vi "CmdExe.Get Processes with Kill Option.vi"(6 "Kill Only 1 Instance":bool=TRUE, 7 "Name Contains":bool, 8 "Error In":errorcluster, 9 "Kill Task":bool, 10 "Process Name":string) -> (0 "Error Out":errorcluster, 1 "Task Killed":bool, 2 "Tasks":string[][](table), 3 "Is Running":bool)   [LabVIEW 2024]
uses:
  <vilib>/Utility/error.llb/Trim Whitespace One-Sided.vi
  <vilib>/KATE/Strings/String Utils.lvlib
panel:
  in  "Tab Control":enum32{"Table", "STDIO"}(tab)
  out "standard output":string
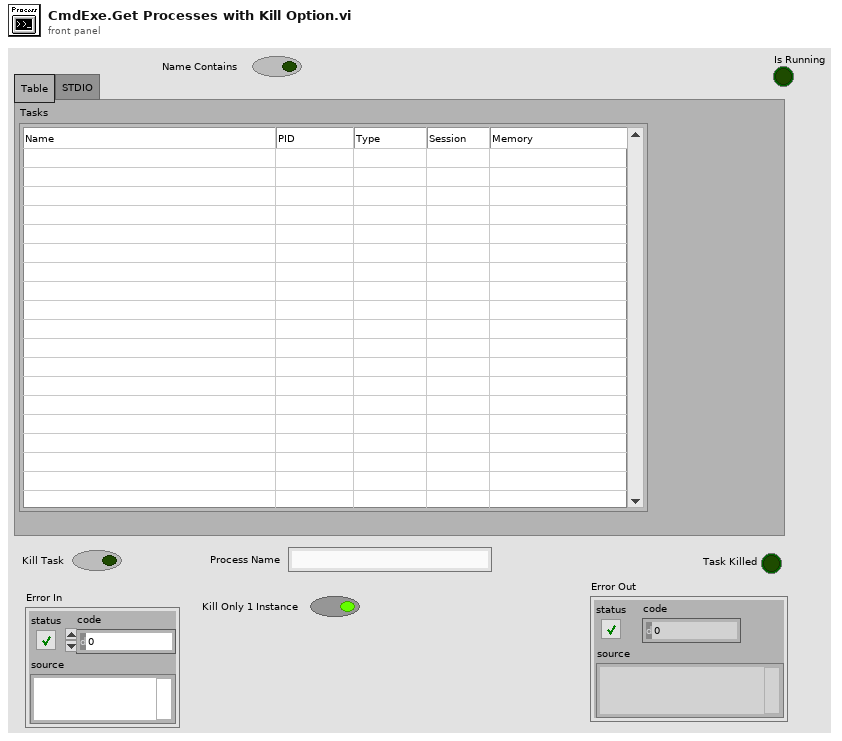
[diagram p1: front panel]
types:
  T1 = cluster{"Stdout":string, "Tasks":string[][], "Index":i32, "PIDs":string[]}
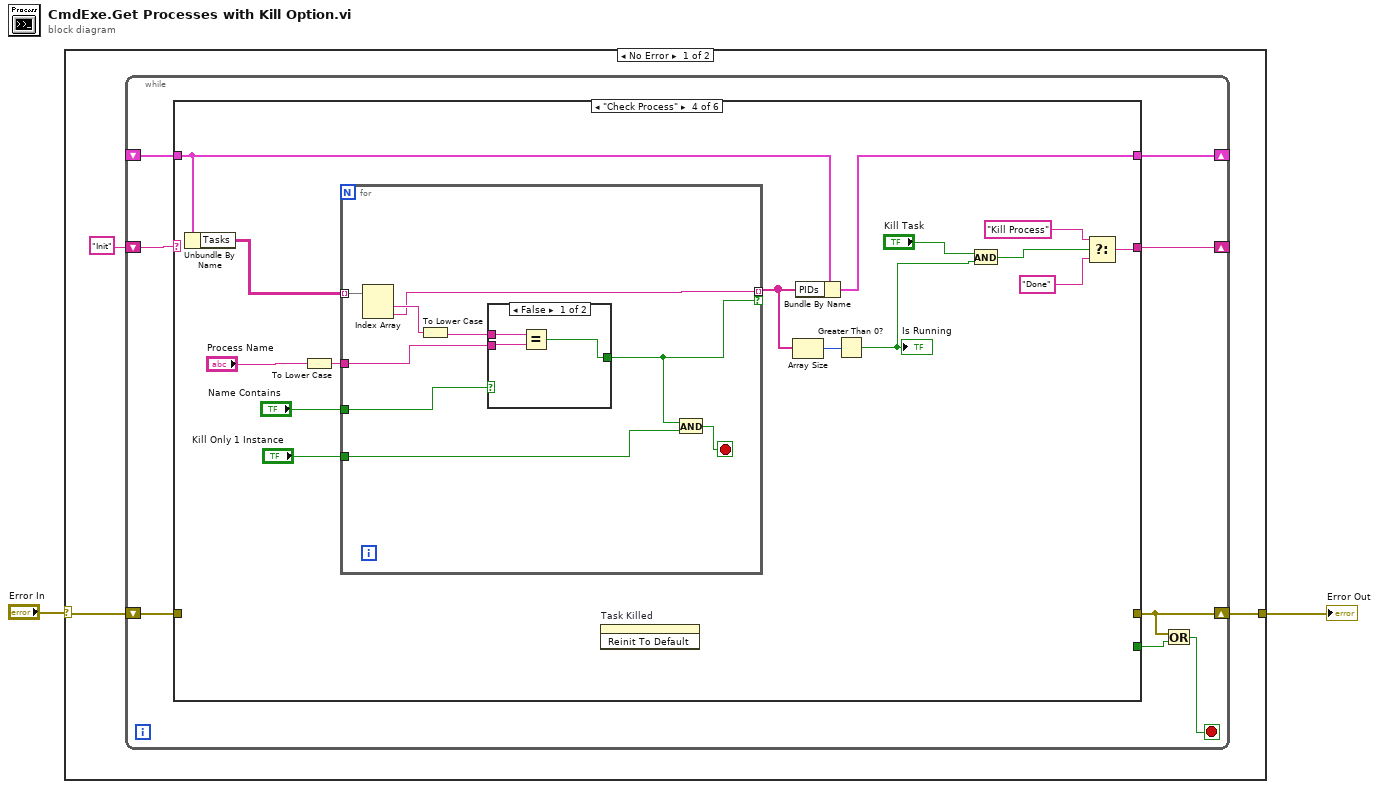
[diagram p0: block diagram]
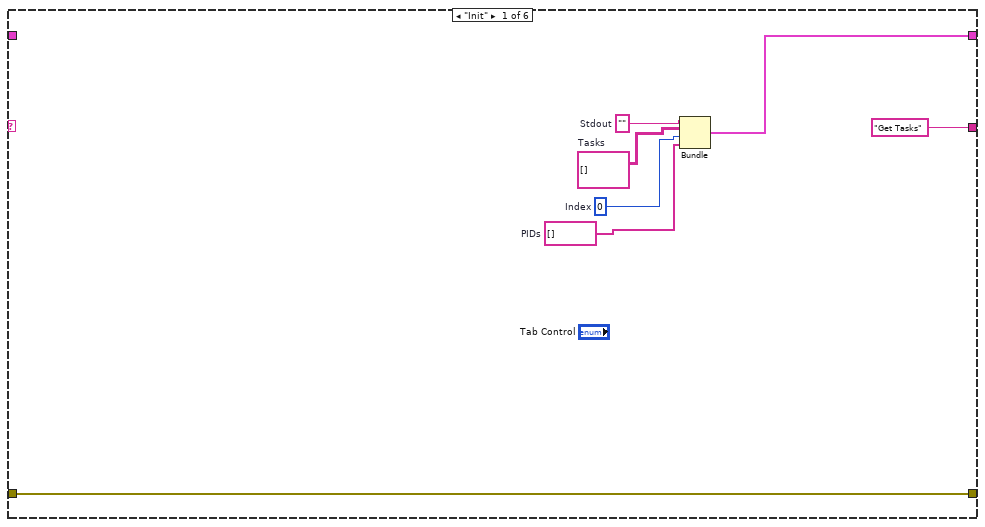
[diagram p2: hidden frame]
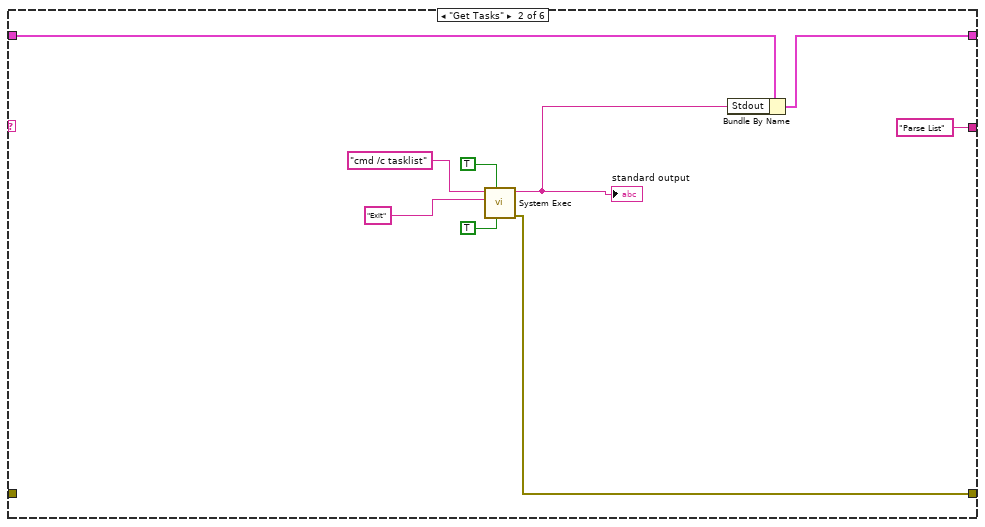
[diagram p3: hidden frame]
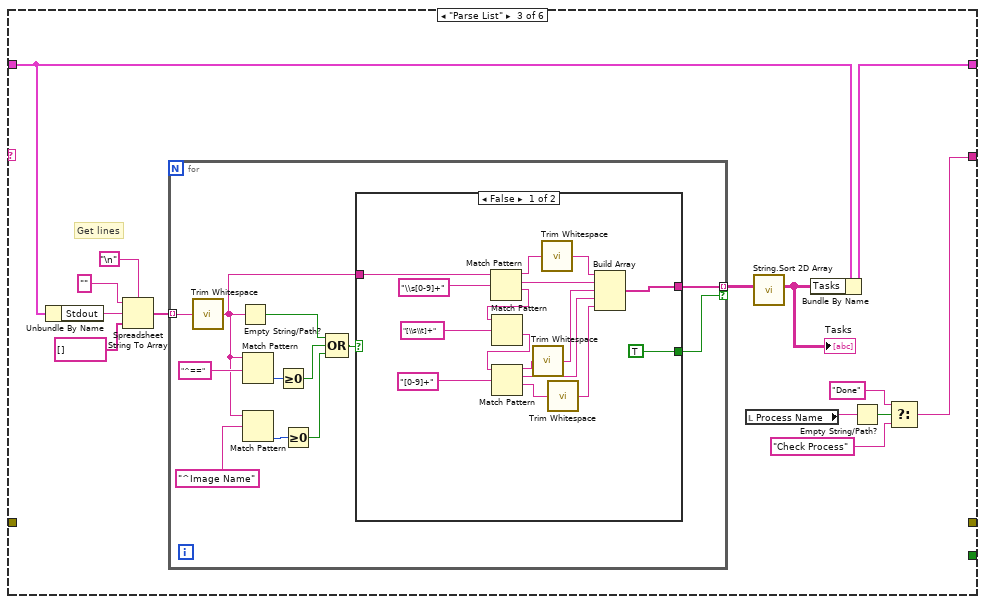
[diagram p4: hidden frame]
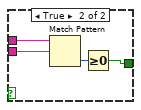
[diagram p6: hidden frame]
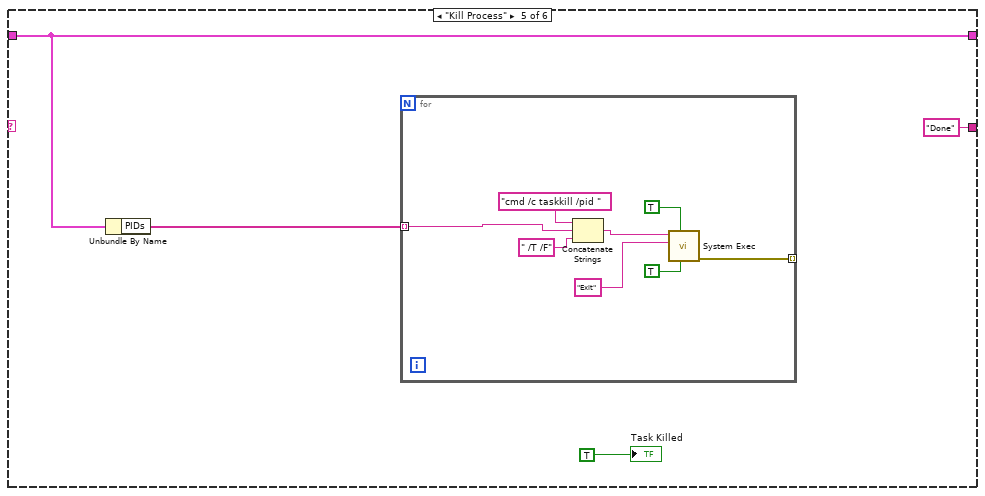
[diagram p7: hidden frame]
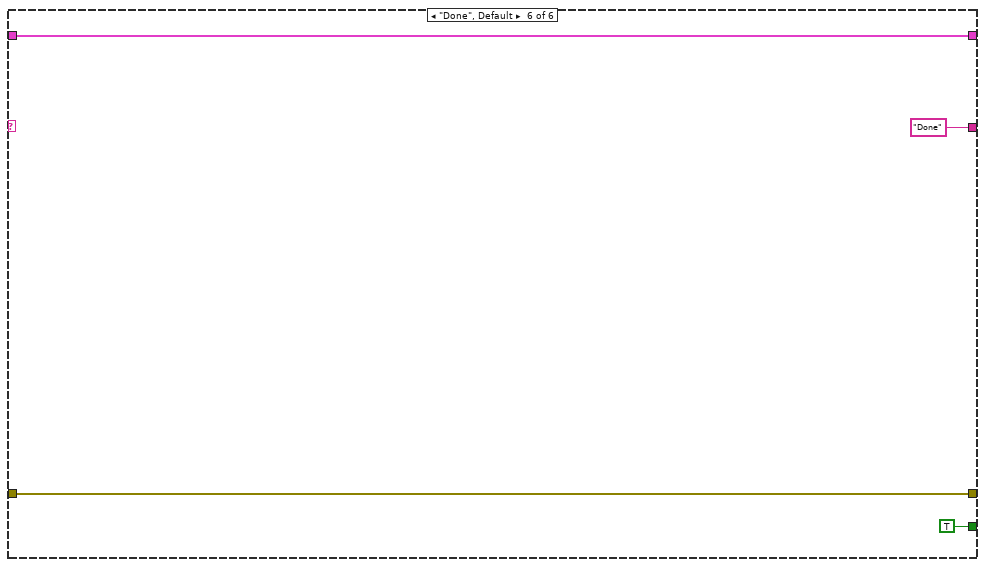
[diagram p8: hidden frame]
diagram:
  n1 = case shown="No Error" "Error In" {
    selector: "Error In" -> [w3 w119]
    tunnel: [w4 w119] -> w2
    frame No Error {
      n2 = while {
        shift-right: [w8] -> _
        shift-left: _ -> [w13]
        shift-right: [w7] -> _
        shift-left: "Init" -> [w9]
        shift-right: [w11] -> w4
        shift-left: w3 -> [w12]
        stop <- w10 stop-if-true
        n3 = case shown="\"Check Process\"" w9 {
          tunnel: w13 -> [_ w28 w41 w85 w105 w118]
          tunnel: w12 -> [w20 _ _ _ _ w116]
          tunnel: [w20 w23 _ _ _ w116] -> w11
          tunnel: [w18 w27 w43 w84 w105 w118] -> w8
          tunnel: ["Get Tasks" "Parse List" w30 w81 "Done" "Done"] -> w7
          tunnel: [_ _ _ _ _ TRUE] -> w6
          frame "Init" {
            w14 = string[] []  # PIDs
            w15 = 0  # Index
            w16 = string[][] []  # Tasks
            w19 = ""  # Stdout
            n4 = Bundle("Stdout"=w19, "Tasks"=w16, "Index"=w15, "PIDs"=w14) -> (w18:T1)  [unwired: 1 in]
          }
          frame "Get Tasks" {
            n5 = call <vilib>:"System Exec.vi"("run minimized? (F)"=TRUE, "wait until completion? (T)"=TRUE, "standard input"="Exit", "command line"="cmd /c tasklist" ("name or relative path")) -> ("error out"=w23:errorcluster, "standard output"=w24:string)  [unwired: 4 in, 2 out]
            "standard output" <- w24
            n6 = Bundle By Name(cluster=w28, "Stdout"=w24) -> (w27:T1)
          }
          frame "Parse List" {
            # "Get lines"
            n7 = Unbundle By Name(w41) -> ("Stdout"=w40:string)
            n8 = Spreadsheet String To Array(delimiter (Tab)="\n", format string="", spreadsheet string=w40, array type (2D Dbl)=string[] [] ("Tasks")) -> (array=w38:string[])
            n9 = for {
              tunnel: w38 -> [w55] mode=indexing
              tunnel: [w49] -> w36 mode=indexing if=w48
              n10 = call <vilib>:"Trim Whitespace.vi"("string"=w55) -> ("trimmed string"=w44:string)  [unwired: 1 in]
              n11 = Empty String/Path?(string/path=w44) -> (empty?=w51:bool)
              n12 = Match Pattern(string=w44, regular expression="^==" ("delimiter (Tab)")) -> (offset past match=w53:i32)  [unwired: 1 in, 3 out]
              n13 = Match Pattern(string=w44, regular expression="^Image Name" ("delimiter (Tab)")) -> (offset past match=w46:i32)  [unwired: 1 in, 3 out]
              n14 = Greater Or Equal To 0?(x=w53) -> (x >= 0?=w52:bool)
              n15 = Greater Or Equal To 0?(x=w46) -> (x >= 0?=w45:bool)
              n16 = Compound Arithmetic op=OR(w51, w52, w45) -> (w50:bool)
              n17 = case shown="False" w50 {
                tunnel: w44 -> [w71 _]
                tunnel: [w68 _] -> w49
                tunnel: [TRUE _] -> w48
                frame False {
                  n18 = Match Pattern(string=w71, regular expression="\\s[0-9]+" ("delimiter (Tab)")) -> (before substring=w58:string, match substring=w62:string, after substring=w70:string)  [unwired: 1 in, 1 out]
                  n19 = Match Pattern(string=w70, regular expression="[\\s\\t]+" ("delimiter (Tab)")) -> (after substring=w69:string)  [unwired: 1 in, 3 out]
                  n20 = Match Pattern(string=w69, regular expression="[0-9]+" ("delimiter (Tab)")) -> (before substring=w57:string, match substring=w61:string, after substring=w63:string)  [unwired: 1 in, 1 out]
                  n21 = call <vilib>:"Trim Whitespace.vi"("string"=w57) -> ("trimmed string"=w56:string)  [unwired: 1 in]
                  n22 = call <vilib>:"Trim Whitespace.vi"("string"=w58) -> ("trimmed string"=w59:string)  [unwired: 1 in]
                  n23 = call <vilib>:"Trim Whitespace.vi"("string"=w63) -> ("trimmed string"=w60:string)  [unwired: 1 in]
                  n24 = Build Array(w59, w62, w56, w61, w60) -> (w68:string[])
                }
                frame True {
                }
              }
            }
            n25 = local read "Process Name"() -> (w33:string)
            n26 = call <vilib>:"String.Sort 2D Array.vi"("Array In"=w36) -> ("Array Out"=w35:string[][])  [unwired: 9 in, 1 out]
            "Tasks" <- w35
            n27 = Bundle By Name(cluster=w41, "Tasks"=w35) -> (w43:T1)
            n28 = Empty String/Path?(string/path=w33) -> (empty?=w34:bool)
            n29 = Select(t="Done", s=w34, f="Check Process") -> (s? t:f=w30:string)
          }
          frame "Check Process" {
            n30 = Unbundle By Name(w85) -> ("Tasks"=w79:string[][])
            n31 = To Lower Case(string="Process Name") -> (all lower case string=w86:string)
            n32 = for {
              tunnel: w86 -> [w95]
              tunnel: w79 -> [w94] mode=indexing
              tunnel: [w91] -> w76 mode=indexing if=w87
              tunnel: "Kill Only 1 Instance" -> [w89]
              tunnel: "Name Contains" -> [w88]
              stop <- w90 stop-if-true
              n33 = Index Array(array=w94) -> (element #1=w93:string, element #2=w91:string)  [unwired: 2 in]
              n34 = To Lower Case(string=w93) -> (all lower case string=w92:string)
              n35 = case shown="False" w88 {
                tunnel: w95 -> [w97 w102]
                tunnel: w92 -> [w98 w101]
                tunnel: [w96 w99] -> w87
                frame False {
                  n36 = Equal?(x=w98, y=w97) -> (x = y?=w96:bool)
                }
                frame True {
                  n37 = Match Pattern(string=w101, regular expression=w102) -> (offset past match=w100:i32)  [unwired: 1 in, 3 out]
                  n38 = Greater Or Equal To 0?(x=w100) -> (x >= 0?=w99:bool)
                }
              }
              n39 = And(x=w87, y=w89) -> (x .and. y?=w90:bool)
            }
            n40 = invoke on="Task Killed" class="Bool (strict)" method="Reinit To Default"() -> ()  [unwired: 3 in, 3 out]
            n41 = Array Size(array=w76) -> (size(s)=w75:i32)
            n42 = Bundle By Name(cluster=w85, "PIDs"=w76) -> (w84:T1)
            n43 = Greater Than 0?(x=w75) -> (x > 0?=w73:bool)
            "Is Running" <- w73
            n44 = And(x="Kill Task", y=w73) -> (x .and. y?=w72:bool)
            n45 = Select(t="Kill Process", s=w72, f="Done") -> (s? t:f=w81:string)
          }
          frame "Kill Process" {
            n46 = Unbundle By Name(w105) -> ("PIDs"=w104:string[])
            n47 = for {
              tunnel: w104 -> [w114] mode=indexing
              tunnel: [w107] -> _ mode=indexing
              n48 = Concatenate Strings("cmd /c taskkill /pid " ("name or relative path"), w114, " /T /F" ("name or relative path")) -> (w109:string)
              n49 = call <vilib>:"System Exec.vi"("run minimized? (F)"=TRUE, "wait until completion? (T)"=TRUE, "standard input"="Exit", "command line"=w109) -> ("error out"=w107:errorcluster)  [unwired: 4 in, 3 out]
            }
            "Task Killed" <- TRUE ("Task Killed")
          }
          frame "Done", Default {
          }
        }
        n50 = Or(x=w11, y=w6) -> (x .or. y?=w10:bool)
      }
    }
    frame Error {
    }
  }
  "Error Out" <- w2
